vi "Msq DeQ.vi"(8 "error in (no error)":errorcluster) -> (0 "error out":errorcluster, 3 "Data":variant, 7 "Module Action":T1)   [LabVIEW 2021, in "Network.lvlib"]
uses:
  Network.lvlib
  Private Controls/Module Action.ctl
  Private Controls/Q Control.ctl
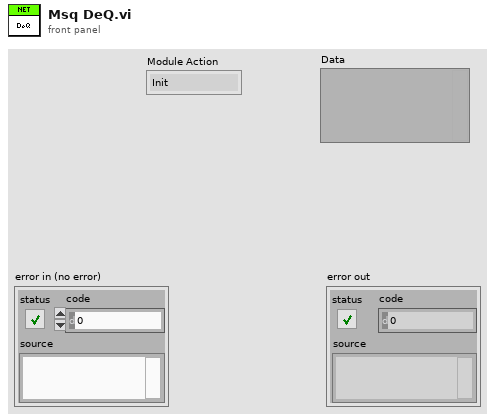
[diagram p1: front panel]
types:
  T1 = typedef "Network.lvlib/Module Action.ctl" = enum16{"Init", "Error", "Close", "PreUUT", "Test Execution", "PostUUT"}
  T2 = typedef "Network.lvlib/Q Control.ctl" = enum16{"Obtain", "Get", "Release"}
  T3 = typedef "EOL Controller.lvlib/Q Msg Dataset.ctl" = cluster{"Module Action":T4, "Data":variant}
  T4 = typedef "EOL Controller.lvlib/Module Action.ctl" = enum16{"Init", "Error", "Close", "PreUUT", "Test Execution", "PostUUT"}
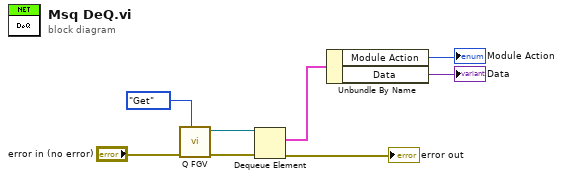
[diagram p0: block diagram]
diagram:
  n1 = call "Q FGV.vi"("Q Control"=Q_Control."Get", "error in (no error)"="error in (no error)") -> ("error out"=w6:errorcluster, "queue out"=w5:refnum<queue>)  [unwired: 8 in]
  n2 = Dequeue Element(queue=w5, error in (no error)=w6) -> (element=w4:T3, error out=→"error out":errorcluster)  [unwired: 1 in, 2 out]
  n3 = Unbundle By Name(w4) -> ("Module Action"=→"Module Action":T4, "Data"=→"Data":variant)
